vi "Retrieve All.vi"(7 "scope":T3, 8 "error in (no error)":errorcluster, 11 "error list <top>":variant) -> (0 "error out":errorcluster, 2 "error list content":cluster{"properties":T1, "errors":T2[]}[](array[cluster]), 3 "error list <top> dup":variant)   [LabVIEW 2017]
uses:
  Scope.ctl
  Error Code File Properties.ctl
  Error File Management/Controls/NI Error.ctl
  Error File Management/Error File Management.lvlib
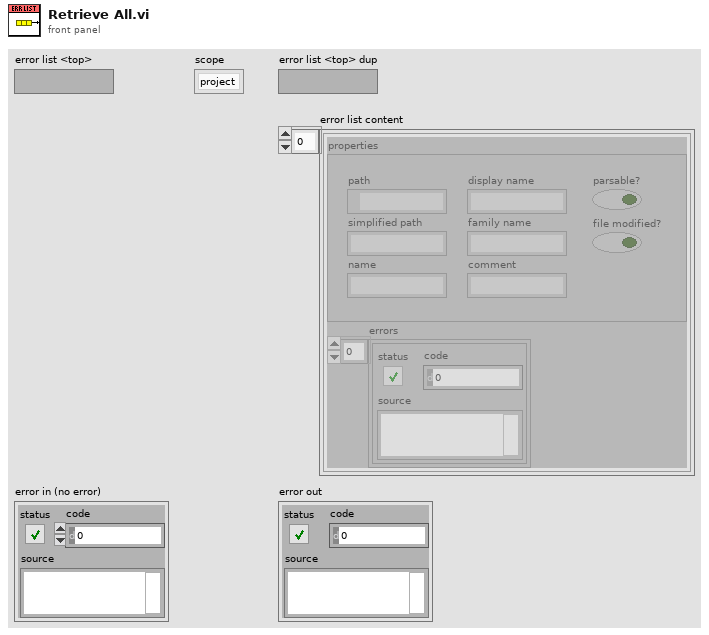
[diagram p1: front panel]
types:
  T1 = typedef "Error Code File Properties.ctl" = cluster{"path":path, "simplified path":string, "name":string, "display name":string, "family name":string, "comment":string, "parsable?":bool, "file modified?":bool}
  T2 = typedef "Error File Management.lvlib/NI Error.ctl" = errorcluster
  T3 = typedef "Scope.ctl" = enum16{"project", "global"}
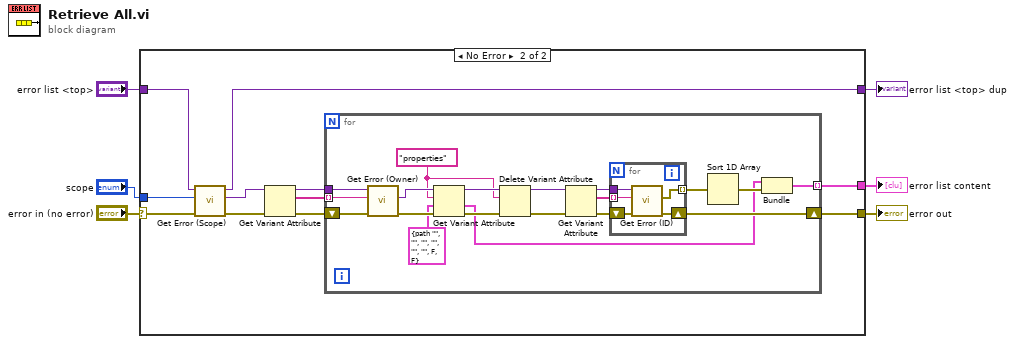
[diagram p0: block diagram]
diagram:
  n1 = case shown="No Error" "error in (no error)" {
    selector: "error in (no error)" -> [w8 w12]
    tunnel: "scope" -> [_ w19]
    tunnel: [w8 w13] -> w4
    tunnel: "error list <top>" -> [w7 w11]
    tunnel: [w7 w10] -> w2
    tunnel: [_ w9] -> w1
    frame Error {
    }
    frame No Error {
      n2 = call "Get Error (Scope).vi"("error in (no error)"=w12, "scope"=w19, "error list <top>"=w11) -> ("error out"=w14:errorcluster, "error list <scope>"=w16:variant, "error list <top> dup"=w10:variant)  [unwired: 5 in, 1 out]
      n3 = Get Variant Attribute(Variant=w16, error in=w14) -> (duplicate Variant=w17:variant, names=w18:string[], error out=w15:errorcluster)  [unwired: 2 in, 1 out]
      n4 = for {
        shift-right: [w34] -> w13
        shift-left: w15 -> [w37]
        tunnel: w18 -> [w33] mode=indexing
        tunnel: w17 -> [w36]
        tunnel: [w20] -> w9 mode=indexing
        w24 = "properties" ("name")
        n5 = call "Get Error (Owner).vi"("error in (no error)"=w37, "owner"=w33, "error list <scope>"=w36) -> ("error out"=w35:errorcluster, "error list <owner>"=w26:variant)  [unwired: 5 in, 2 out]
        n6 = Get Variant Attribute(Variant=w26, name=w24, default value (empty Variant)=T1 {"path"=path "", "simplified path"="", "name"="", "display name"="", "family name"="", "comment"="", "parsable?"=FALSE, "file modified?"=FALSE} ("properties"), error in=w35) -> (duplicate Variant=w25:variant, value=w22:T1, error out=w27:errorcluster)  [unwired: 1 out]
        n7 = Delete Variant Attribute(4:w27, 6:w24, 7:w25) -> (0:w29:errorcluster, 3:w28:variant)  [unwired: 1 out]
        n8 = Get Variant Attribute(Variant=w28, error in=w29) -> (duplicate Variant=w31:variant, names=w30:string[], error out=w32:errorcluster)  [unwired: 2 in, 1 out]
        n9 = for {
          shift-right: [w42] -> w34
          shift-left: w32 -> [w43]
          tunnel: w30 -> [w40] mode=indexing
          tunnel: [w39] -> w21 mode=indexing
          tunnel: w31 -> [w41]
          n10 = call "Get Error (ID).vi"("error in (no error)"=w43, "ID"=w40, "error list <owner>"=w41) -> ("error out"=w42:errorcluster, "error"=w39:T2)  [unwired: 4 in, 3 out]
        }
        n11 = Sort 1D Array(array=w21) -> (sorted array=w38:T2[])
        n12 = Bundle("properties"=w22, w38) -> (w20:cluster{"properties":T1, T2[]})  [unwired: 1 in]
      }
    }
  }
  "error out" <- w4
  "error list <top> dup" <- w2
  "error list content" <- w1
